vi "Aplicacao_atual_global_adq.vi"() -> ()   [LabVIEW 2019]
panel:
  out "APLICACAO ATUAL":string
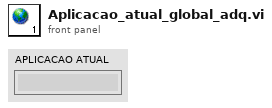
[diagram p1: front panel]
diagram:
